vi "Create Database.vi"(8 "error in (no error)":errorcluster, 11 "User Interface in":refnum<class "User Interface.lvclass">) -> (0 "error out":errorcluster, 3 "User Interface out":refnum<class "User Interface.lvclass">)   [LabVIEW 2020, in "User Interface.lvlib" / "User Interface.lvclass"]
uses:
  User Interface.lvclass
  User Interface.lvclass/User Interface.ctl
  Paquetes Disponibles Messages/Database Path Msg/Database Path Msg.lvclass/Database Path Msg.ctl
  <vilib>/ActorFramework/Message Enqueuer/Message Enqueuer.lvclass/Message Enqueuer.ctl
  <vilib>/drjdpowell/SQLite Library/SQL Connection/Open (path).vi
  <vilib>/ActorFramework/Message Enqueuer/Enqueue.vi
  <vilib>/drjdpowell/SQLite Library/SQL Connection/Open (string).vi
  Paquetes Disponibles Messages/Database Path Msg/Database Path Msg.lvclass
  C:/Program Files (x86)/National Instruments/LabVIEW 2020/vi.lib/ActorFramework/Message/Message.lvclass
  <vilib>/ActorFramework/Message Priority Queue/Priority Enqueue.vi
  <vilib>/AdvancedString/Path To Command Line String.vi
  <vilib>/drjdpowell/SQLite Library/SQL Connection/Execute SQL (No results).vi
  <vilib>/drjdpowell/SQLite Library/SQL Connection/Connection.lvclass
  <vilib>/drjdpowell/SQLite Library/SQLite.lvlib
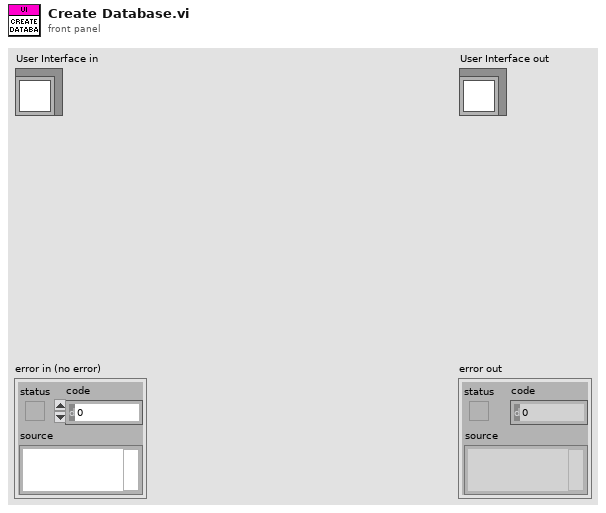
[diagram p1: front panel]
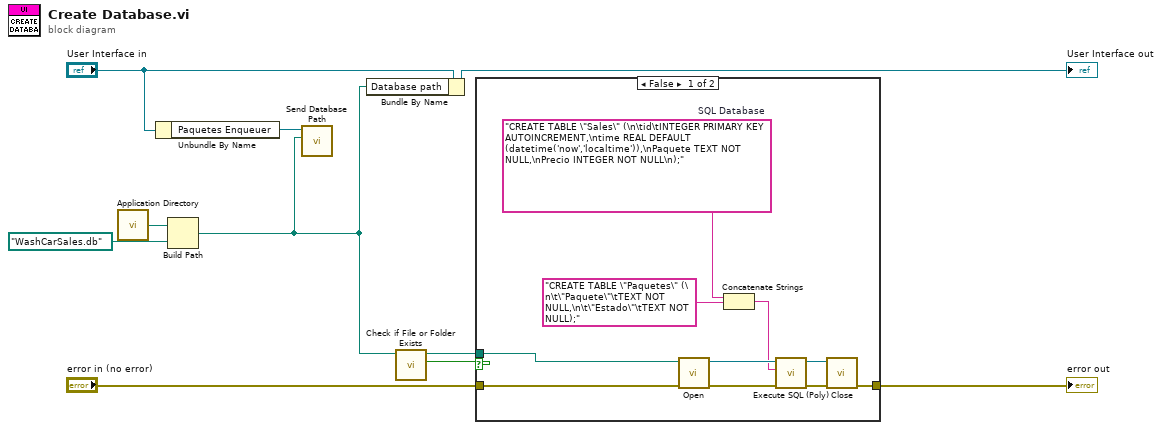
[diagram p0: block diagram]
diagram:
  n1 = call <vilib>:"Application Directory.vi"() -> ("Application Directory"=w8:path)
  n2 = Unbundle By Name("User Interface in") -> ("Paquetes Enqueuer"=w3:refnum<class "Message Enqueuer.lvclass">)
  n3 = Build Path(base path=w8, name or relative path=path "WashCarSales.db") -> (appended path=w1:path)
  n4 = call "Send Database Path.vi"("Database path"=w1, "Message Enqueuer"=w3) -> ()  [unwired: 8 in, 2 out]
  n5 = Bundle By Name(cluster="User Interface in", "Database path"=w1) -> (→"User Interface out":refnum<class "User Interface.lvclass">)
  n6 = call <vilib>:"Check if File or Folder Exists.vi"("path"=w1) -> ("file or folder exists?"=w10:bool, "dup path"=w9:path)  [unwired: 8 in, 1 out]
  n7 = case shown="False" w10 {
    tunnel: [w18 w21] -> w5
    tunnel: w9 -> [w17 _]
    tunnel: "error in (no error)" -> [w14 w21]
    frame False {
      w13 = "CREATE TABLE \"Sales\" (\n\tid\tINTEGER PRIMARY KEY AUTOINCREMENT,\ntime REAL DEFAULT (datetime('now','localtime')),\nPaquete TEXT NOT NULL,\nPrecio INTEGER NOT NULL\n);"  # SQL Database
      n8 = call-poly <vilib>:"Open.vi"("error in (no error)"=w14, "db file"=w17) -> ("error out"=w20:errorcluster, "SQLite Connection"=w16:refnum<class "Connection.lvclass">)  [unwired: 8 in]
      n9 = Concatenate Strings(w13, "CREATE TABLE \"Paquetes\" (\n\t\"Paquete\"\tTEXT NOT NULL,\n\t\"Estado\"\tTEXT NOT NULL);") -> (w11:string)
      n10 = call-poly <vilib>:"Execute SQL (Poly).vi"("error in (no error)"=w20, "SQL"=w11, "SQLite Connection in"=w16) -> ("error out"=w19:errorcluster, "SQLite Connection"=w15:refnum<class "Connection.lvclass">)  [unwired: 7 in]
      n11 = call-dynamic "Close.vi"("error in (no error)"=w19, "SQLite Connection in"=w15) -> ("error out"=w18:errorcluster)  [unwired: 9 in]
    }
    frame True {
    }
  }
  "error out" <- w5
